vi "RotateZ.vi"(1 "theta":dbl) -> (0 "rotation matrix":T1)   [LabVIEW 2017, in "NI_Kinematics.lvlib"]
uses:
  <vilib>/robotics/Kinematics/NI_Kinematics.lvlib
  <vilib>/Analysis/Matrix/Datatypes/RealMatrix.ctl
  <vilib>/Analysis/Matrix/NI_Matrix.lvlib
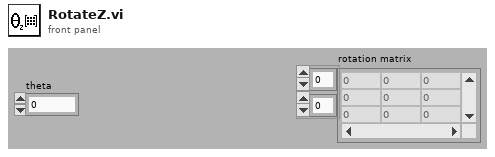
[diagram p1: front panel]
types:
  T1 = typedef "NI_Matrix.lvlib/RealMatrix.ctl" = dbl[][]
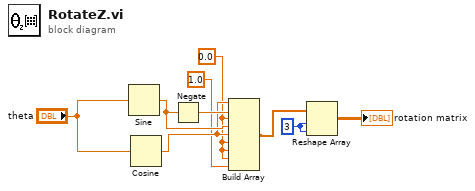
[diagram p0: block diagram]
diagram:
  w2 = 0.0
  w9 = 3 ("number of rows")
  n1 = Sine(x="theta") -> (sin(x)=w6:dbl)
  n2 = Cosine(x="theta") -> (cos(x)=w4:dbl)
  n3 = Negate(x=w6) -> (-x=w5:dbl)
  n4 = Build Array(w4, w5, w2, w6, w4, w2, w2, w2, 1.0) -> (w1:dbl[])
  n5 = Reshape Array(w1, w9, w9) -> (→"rotation matrix":dbl[][])
